vi "Create DO Channel.vi"(6 "index":i32, 8 "error in":errorcluster, 9 "default value":bool, 10 "name":string, 11 "DO channel in":refnum<class "DO Channel.lvclass">) -> (0 "error out":errorcluster, 3 "DO channel out":refnum<class "DO Channel.lvclass">)   [LabVIEW 2020, in "Scan Engine Scripting.lvlib" / "DO Channel.lvclass"]
uses:
  DO Channel.lvclass
  Channel/Type.ctl
  Channel/Channel.lvclass
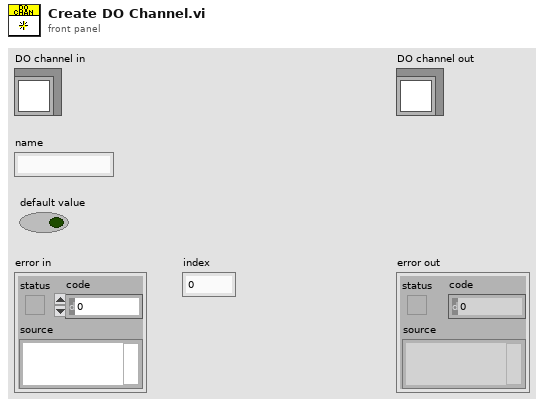
[diagram p1: front panel]
types:
  T1 = typedef "Scan Engine Scripting.lvlib/Channel.lvclass/Type.ctl" = enum16{"Input", "Output"}
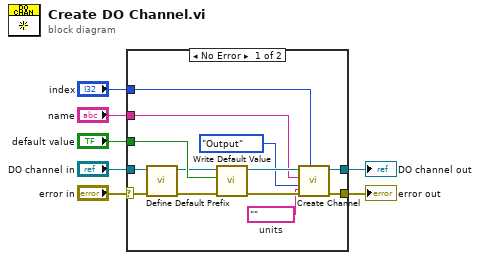
[diagram p0: block diagram]
diagram:
  n1 = case shown="No Error" "error in" {
    selector: "error in" -> [w9 w22]
    tunnel: "name" -> [w17 _]
    tunnel: "default value" -> [w16 _]
    tunnel: [w15 w22] -> w5
    tunnel: [w14 w21] -> w4
    tunnel: "index" -> [w13 _]
    tunnel: "DO channel in" -> [w12 w21]
    frame No Error {
      w8 = ""  # units
      n2 = call-dynamic "Define Default Prefix.vi"("error in (no error)"=w9, "DO Channel in"=w12) -> ("error out"=w11:errorcluster, "DO Channel out"=w10:refnum<class "DO Channel.lvclass">)  [unwired: 8 in]
      n3 = call-dynamic "Write Default Value.vi"("error in"=w11, "default value"=w16, "digital channel in"=w10) -> ("error out"=w20:errorcluster, "digital channel out"=w19:refnum<class "DO Channel.lvclass">)  [unwired: 7 in]
      n4 = call-dynamic "Create Channel.vi"("units"=w8, "index"=w13, "error in"=w20, "type"=Type."Output", "name"=w17, "channel in"=w19) -> ("error out"=w15:errorcluster, "channel out"=w14:refnum<class "DO Channel.lvclass">)  [unwired: 4 in]
    }
    frame Error {
    }
  }
  "error out" <- w5
  "DO channel out" <- w4
